vi "FA_Update_Events.vi"(8 "error in (no error)":errorcluster, 11 "Attendance XML":string) -> (0 "error out":errorcluster)   [LabVIEW 2013, in "FA_FIRST.lvlib"]
uses:
  FA_FIRST.lvlib
  Backend/source/VI Source/FRCts20_Backend_API/FRCts20_Backend_API_Event.ctl
  Backend/source/VI Source/FRCts20_Backend_API/FRCts20_Backend_API_SW.ctl
  Backend/source/VI Source/FRCts20_Backend_API/FRCts20_Backend_API_Command_EventRoot.ctl
  Backend/source/VI Source/FRCts20_Backend_API/FRCts20_Backend_API_EventRoot.ctl
  Backend/source/VI Source/FRCts20_Backend_API/FRCts20_Backend_API_Command_Event.ctl
  Backend/source/VI Source/FRCts20_Backend_API/FRCts20_Backend_API_EventRoot.vi
  Backend/source/VI Source/FRCts20_Backend_API/FRCts20_Backend_API_Event.vi
  Backend/source/VI Source/FRCts20_Backend_API/FRCts20_Backend_API.lvlib
panel:
  out "Numeric":i32
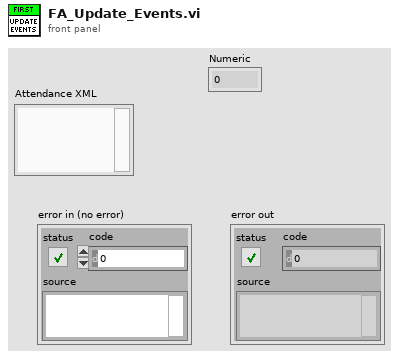
[diagram p1: front panel]
types:
  T1 = typedef "FRCts20_Backend_API.lvlib/FRCts20_Backend_API_EventRoot.ctl" = cluster{"Event":cluster{"Event Index":u32, "Event Name":string, "Start Time":timestamp, "End Time":timestamp, "OpenIssues":u8, "IsLive":bool}[], "APIReturn":string}
  T2 = typedef "FRCts20_Backend_API.lvlib/FRCts20_Backend_API_Command_EventRoot.ctl" = string
  T3 = typedef "FRCts20_Backend_API.lvlib/FRCts20_Backend_API_Command_Event.ctl" = string
  T4 = typedef "FRCts20_Backend_API.lvlib/FRCts20_Backend_API_Event.ctl" = cluster{"Event Index":u32, "Name":string, "Start Time":timestamp, "End Time":timestamp, "Teams":cluster{"Team Index":u32, "Team Number":u32, "Requests":cluster{"Request Number":u32, "Description":string}[], "Has Open Issue":bool}[], "SWType":T5, "APIReturn":string}
  T5 = typedef "FRCts20_Backend_API.lvlib/FRCts20_Backend_API_SW.ctl" = string
  T6 = cluster{"Event Index":u32, "Event Name":string, "Start Time":timestamp, "End Time":timestamp, "OpenIssues":u8, "IsLive":bool}[]
  T7 = cluster{"Team Index":u32, "Team Number":u32, "Requests":cluster{"Request Number":u32, "Description":string}[], "Has Open Issue":bool}[]
  T8 = cluster{"Team Index":u32, "Team Number":u32, "Requests":cluster{"Request Number":u32, "Description":string}[], "Has Open Issue":bool}
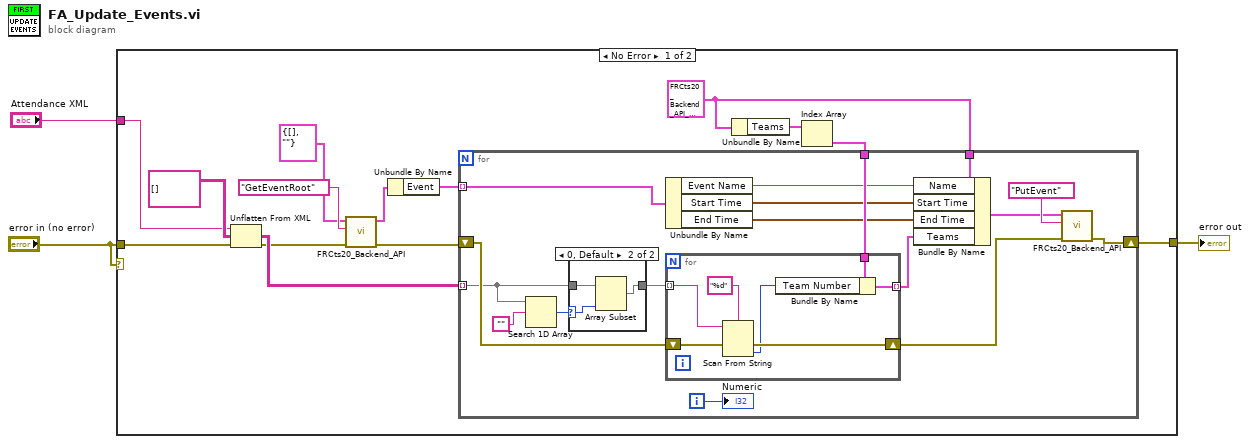
[diagram p0: block diagram]
diagram:
  n1 = case shown="No Error" "error in (no error)" {
    tunnel: "error in (no error)" -> [w15 _]
    tunnel: "Attendance XML" -> [w16 _]
    tunnel: [w10 _] -> w1
    frame No Error {
      w13 = T4 {"Event Index"=0, "Name"="", "Start Time"=timestamp(0 s since 1904-01-01), "End Time"=timestamp(0 s since 1904-01-01), "Teams"=[], "SWType"="", "APIReturn"=""} ("Event In")
      n2 = Unflatten From XML(xml string=w16, type=string[][] [] ("transposed array"), error in (no error)=w15) -> (value=w14:string[][], error out=w9:errorcluster)
      n3 = call-poly "FRCts20_Backend_API.vi"("error in (no error)"=w9, "Message"=T2 "GetEventRoot", "EventRoot In"=T1 {"Event"=[], "APIReturn"=""}) -> ("error out"=w8:errorcluster, "EventRoot Out"=w5:T1)  [unwired: 6 in, 1 out]
      n4 = Unbundle By Name(w5) -> ("Event"=w4:T6)
      n5 = Unbundle By Name(w13) -> ("Teams"=w12:T7)
      n6 = Index Array(array=w12) -> (element=w11:T8)  [unwired: 1 in]
      n7 = for {
        shift-right: [w26] -> w10
        shift-left: w8 -> [w32]
        tunnel: w13 -> [w34]
        tunnel: w14 -> [w19] mode=indexing
        tunnel: w11 -> [w33]
        tunnel: w4 -> [w31] mode=indexing
        i -> [w22]
        n8 = Search 1D Array(1D array=w19, element="") -> (index of element=w20:i32)  [unwired: 1 in]
        n9 = case shown="0, Default" w20 {
          selector: w20 -> [_ w38]
          tunnel: w19 -> [w35 w37]
          tunnel: [w35 w36] -> w18
          frame -1 {
          }
          frame 0, Default {
            n10 = Array Subset(array=w37, length=w38) -> (w36:string[])  [unwired: 1 in]
          }
        }
        n11 = Unbundle By Name(w31) -> ("Event Name"=w30:string, "Start Time"=w28:timestamp, "End Time"=w27:timestamp)
        n12 = for {
          tunnel: w18 -> [w45] mode=indexing
          tunnel: w33 -> [w44]
          tunnel: [w42] -> w29 mode=indexing
          shift-right: [w40] -> w25
          shift-left: w32 -> [w41]
          n13 = Scan From String(format string="%d", input string=w45, error in=w41) -> (error out=w40:errorcluster, output 1=w39:i32)  [unwired: 2 in, 2 out]
          n14 = Bundle By Name(cluster=w44, "Team Number"=w39) -> (w42:T8)
        }
        n15 = Bundle By Name(cluster=w34, "Name"=w30, "Start Time"=w28, "End Time"=w27, "Teams"=w29) -> (w23:T4)
        n16 = call-poly "FRCts20_Backend_API.vi"("error in (no error)"=w25, "Command"=T3 "PutEvent", "Event In"=w23) -> ("error out"=w26:errorcluster)  [unwired: 6 in, 2 out]
        "Numeric" <- w22
      }
    }
    frame Error {
    }
  }
  "error out" <- w1
